vi "WillHeadingHitObstacles.vi"(7 "Safety offset around edges (m)":dbl=5.0, 9 "Heading":dbl, 10 "Boat":T1 {"North" format="%#_10f"; "East" format="%#_8f"}, 11 "Obstacle.lvclass":refnum<class "Obstacle.lvclass">) -> (2 "Any intersecting obstacles?":bool, 3 "Intersecting obstacles array":bool[](array[boolean]))   [LabVIEW 2013, in "Obstacle.lvclass"]
uses:
  Obstacle.lvclass
  Data/TypeDefs/UTM Location.ctl
  Obstacle.lvclass/Obstacle.ctl
panel:
  in  "error in (no error)":errorcluster
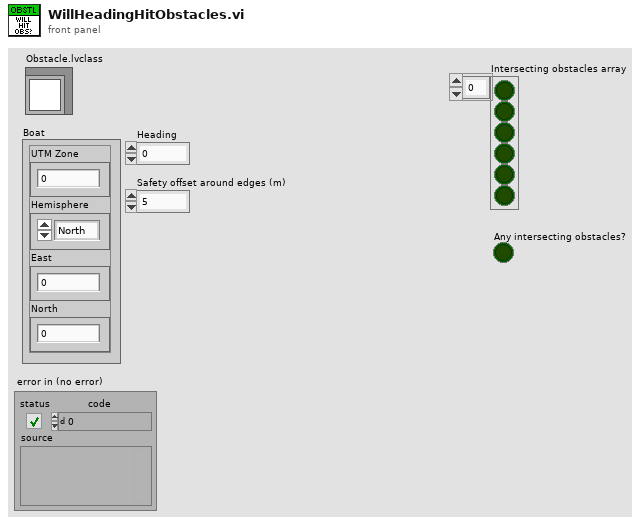
[diagram p1: front panel]
types:
  T1 = typedef "UTM Location.ctl" = cluster{"UTM Zone":dbl, "Hemisphere":enum16{"North", "South"}, "East":dbl, "North":dbl}
  T2 = cluster{"UTM Obstacle Point 2":T1, "UTM Obstacle Point 1":T1}[]
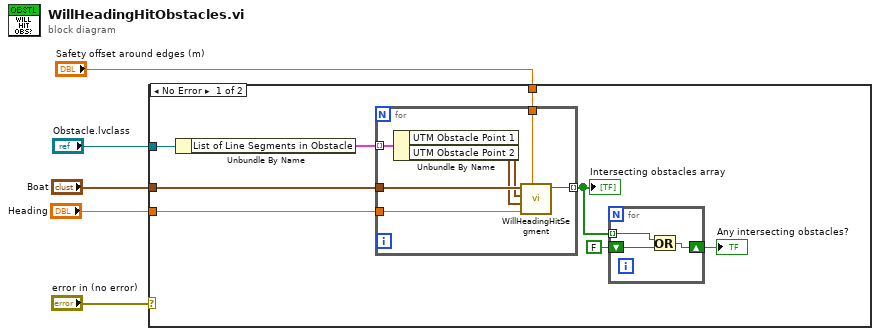
[diagram p0: block diagram]
diagram:
  n1 = case shown="No Error" "error in (no error)" {
    tunnel: "Obstacle.lvclass" -> [w13 _]
    tunnel: "Boat" -> [w11 _]
    tunnel: "Heading" -> [w10 _]
    tunnel: "Safety offset around edges (m)" -> [w9 _]
    frame No Error {
      n2 = Unbundle By Name(w13) -> ("List of Line Segments in Obstacle"=w12:T2)
      n3 = for {
        tunnel: w12 -> [w23] mode=indexing
        tunnel: w11 -> [w22]
        tunnel: w10 -> [w21]
        tunnel: w9 -> [w18]
        tunnel: [w17] -> w8 mode=indexing
        n4 = Unbundle By Name(w23) -> ("UTM Obstacle Point 1"=w20:T1, "UTM Obstacle Point 2"=w19:T1)
        n5 = call "WillHeadingHitSegment.vi"("Safety offset around edges (m)"=w18, "Heading (deg)"=w21, "Segment Point 2"=w19, "Segment Point 1"=w20, "Boat Point"=w22) -> ("Will collide"=w17:bool)  [unwired: 6 in]
      }
      "Intersecting obstacles array" <- w8
      n6 = for {
        tunnel: w8 -> [w15] mode=indexing
        shift-right: [w14] -> w6
        shift-left: FALSE -> [w16]
        n7 = Or(x=w15, y=w16) -> (x .or. y?=w14:bool)
      }
      "Any intersecting obstacles?" <- w6
    }
    frame Error {
    }
  }
